vi "ImageGetElapsedTime.vi"(11 "start time":dbl) -> (3 "time elapsed (s)":dbl)   [LabVIEW 2012, in "Image.lvclass"]
uses:
  classes/Image.lvclass
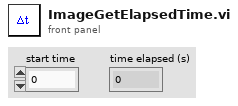
[diagram p1: front panel]
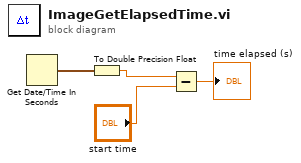
[diagram p0: block diagram]
diagram:
  n1 = Get Date/Time In Seconds() -> (seconds since 1Jan1904=w3:timestamp)
  n2 = To Double Precision Float(number=w3) -> (double precision float=w4:dbl)
  n3 = Subtract(x=w4, y="start time") -> (x-y=→"time elapsed (s)":dbl)
